vi "ReadCAlexFile.vi"(8 "error in (no error)":errorcluster, 10 "ExpData File Path":path, 11 "CAlexData2":refnum<class "CAlexData2.lvclass">) -> (0 "error out":errorcluster, 3 "CAlexData 2":refnum<class "CAlexData2.lvclass">)   [LabVIEW 2015, in "CAlexData2.lvclass"]
uses:
  CAlexData2.lvclass
  CAlex2/CAlex2.lvclass
  CAlex2/TypeDef/LowerBodyDim.ctl
  CAlexData2.lvclass/CAlexData2.ctl
  ExpData/ExpData.lvclass
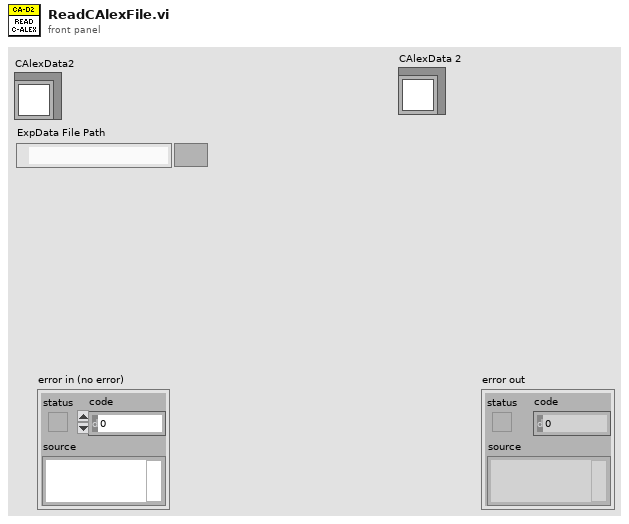
[diagram p1: front panel]
types:
  T1 = typedef "CAlex2.lvclass/LowerBodyDim.ctl" = cluster{"BodyDim(m)":cluster{"ThighLt":dbl, "ShankLt":dbl, "HipWd":dbl}, "BodyWt(kg)":cluster{"Thigh":dbl, "Shank":dbl}, "CuffLoc(m)":cluster{"HipCuffWd":dbl, "HipCuffHt":dbl, "HipCuffFwdShift":dbl, "ThighCuffToKnee":dbl, "ThighCuffDist":dbl, "ShankCuffToKnee":dbl}}
  T2 = cluster{"[0]":dbl, "[1]":dbl, "[2]":dbl, "[3]":dbl, "[4]":dbl, "[5]":dbl}
  T3 = cluster{"array type (2D Dbl)[0]":dbl, "array type (2D Dbl)[1]":dbl, "array type (2D Dbl)[2]":dbl, "array type (2D Dbl)[3]":dbl, "array type (2D Dbl)[4]":dbl, "array type (2D Dbl)[5]":dbl}
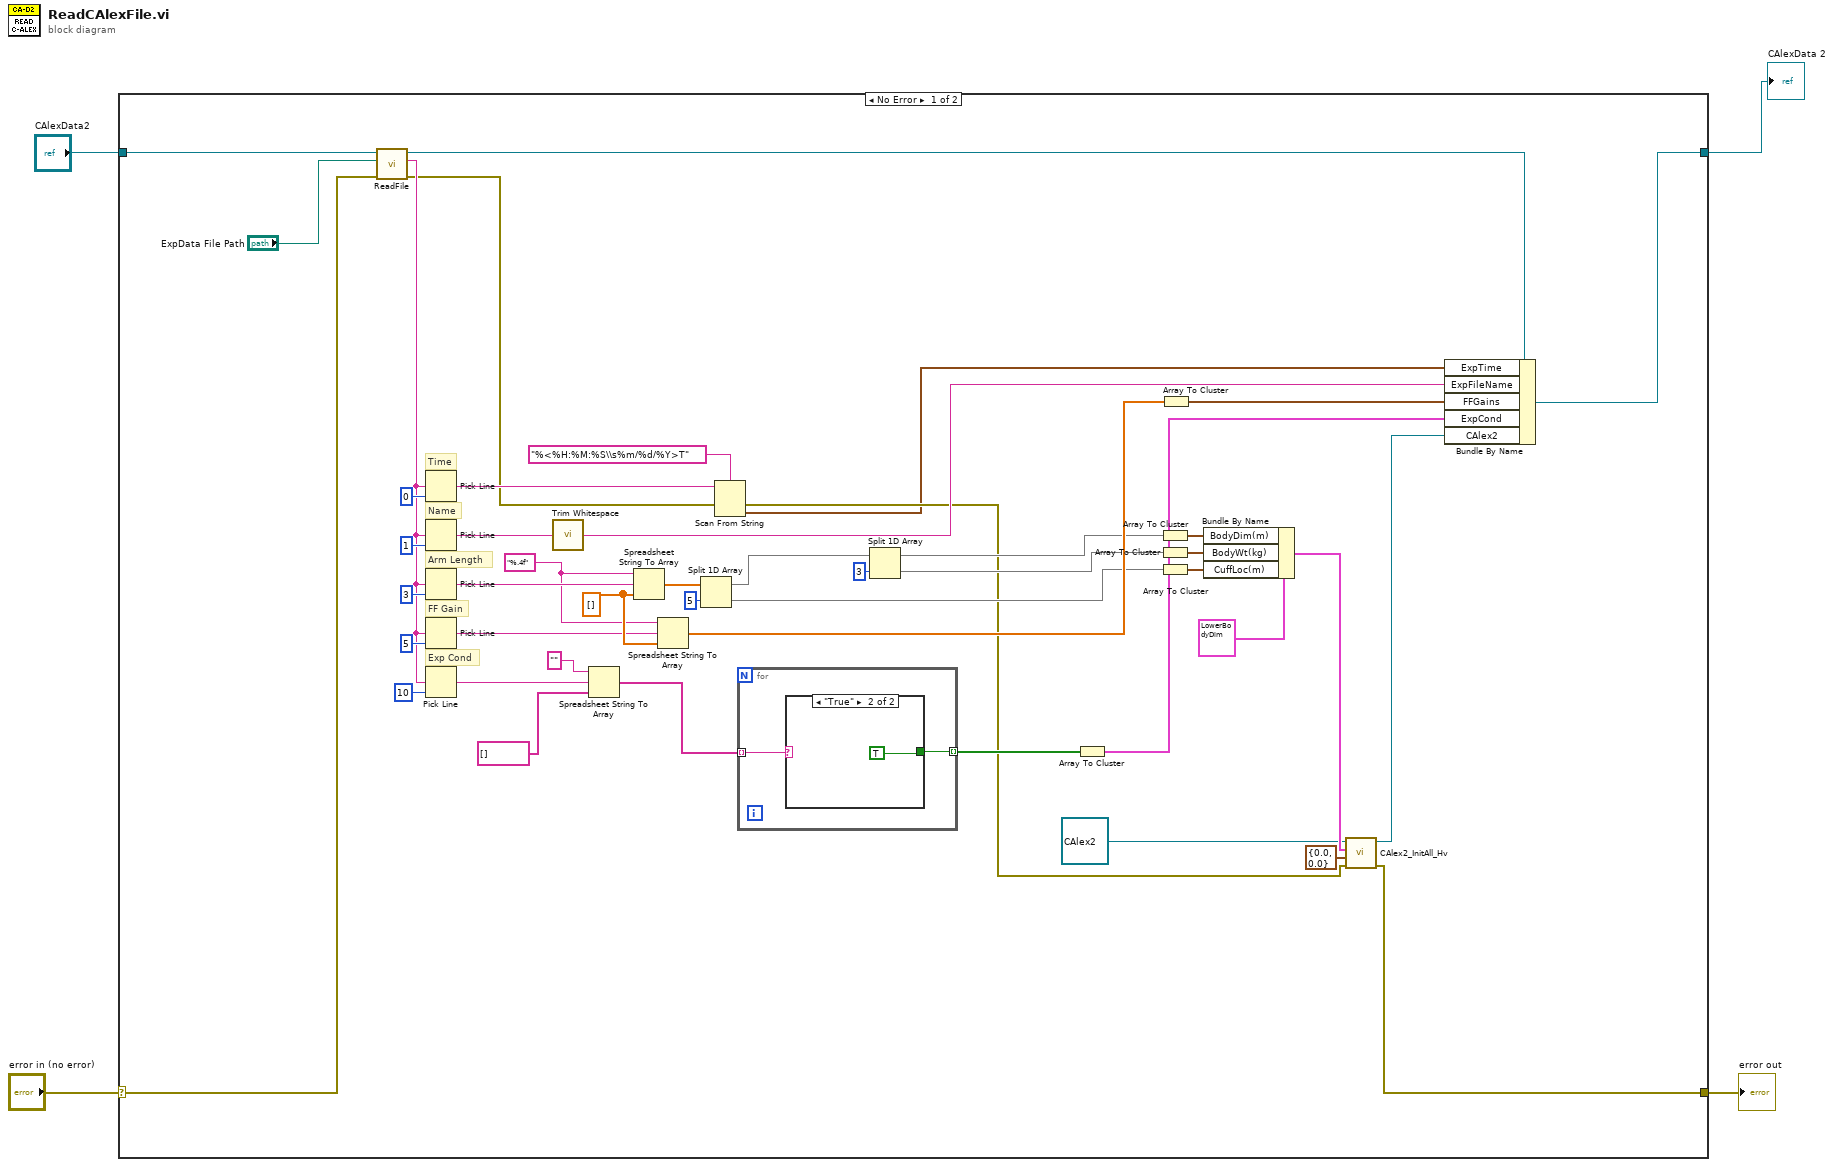
[diagram p0: block diagram]
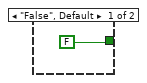
[diagram p2: hidden frame]
diagram:
  n1 = case shown="No Error" "error in (no error)" {
    selector: "error in (no error)" -> [w31 w56]
    tunnel: [w11 w56] -> w3
    tunnel: [w8 w55] -> w1
    tunnel: "CAlexData2" -> [w10 w55]
    frame No Error {
      w35 = "%.4f" ("format (%.3f)")
      w49 = dbl[] [] ("array type (2D Dbl)")
      # "Exp Cond"
      # "FF Gain"
      # "Arm Length"
      # "Name"
      # "Time"
      n2 = call "ReadFile.vi"("error in (no error)"=w31, "ExpData File Path"="ExpData File Path", "ExpData In"=w10) -> ("error out"=w32:errorcluster, "MetaData"=w33:string, "ExpData Out"=w9:refnum<class "CAlexData2.lvclass">)  [unwired: 5 in, 1 out]
      n3 = Pick Line(multi-line string=w33, line index=0) -> (output string=w40:string)  [unwired: 1 in]
      n4 = Pick Line(multi-line string=w33, line index=1) -> (output string=w41:string)  [unwired: 1 in]
      n5 = Pick Line(multi-line string=w33, line index=3) -> (output string=w44:string)  [unwired: 1 in]
      n6 = Pick Line(multi-line string=w33, line index=5) -> (output string=w46:string)  [unwired: 1 in]
      n7 = Pick Line(multi-line string=w33, line index=10) -> (output string=w48:string)  [unwired: 1 in]
      n8 = call <vilib>:"Trim Whitespace.vi"("string"=w41) -> ("trimmed string"=w38:string)  [unwired: 1 in]
      n9 = Spreadsheet String To Array(format string="", spreadsheet string=w48, array type (2D Dbl)=string[] []) -> (array=w21:string[])  [unwired: 1 in]
      n10 = Spreadsheet String To Array(format string=w35, spreadsheet string=w44, array type (2D Dbl)=w49) -> (array=w36:dbl[])  [unwired: 1 in]
      n11 = Spreadsheet String To Array(format string=w35, spreadsheet string=w46, array type (2D Dbl)=w49) -> (array=w30:dbl[])  [unwired: 1 in]
      n12 = Split 1D Array(array=w36, index=5) -> (first subarray=w27:dbl[], second subarray=w24:dbl[])
      n13 = Scan From String(format string="%<%H:%M:%S\\s%m/%d/%Y>T", input string=w40, error in=w32) -> (error out=w12:errorcluster, output 1=w5:timestamp)  [unwired: 2 in, 2 out]
      n14 = for {
        tunnel: w21 -> [w52] mode=indexing
        tunnel: [w51] -> w20 mode=indexing
        n15 = case shown="\"True\"" w52 {
          tunnel: [FALSE TRUE] -> w51
          frame "False", Default {
          }
          frame "True" {
          }
        }
      }
      n16 = Split 1D Array(array=w27, index=3) -> (first subarray=w26:dbl[], second subarray=w25:dbl[])
      n17 = Array To Cluster(array=w20) -> (cluster=w19:cluster{"[0]":bool, "[1]":bool, "[2]":bool})
      n18 = Array To Cluster(array=w26) -> (cluster=w18:cluster{"[0]":dbl, "[1]":dbl, "[2]":dbl})
      n19 = Array To Cluster(array=w25) -> (cluster=w17:cluster{"[0]":dbl, "[1]":dbl})
      n20 = Array To Cluster(array=w24) -> (cluster=w16:T2)
      n21 = Array To Cluster(array=w30) -> (cluster=w29:T3)
      n22 = Bundle By Name(cluster=T1 {"BodyDim(m)"={"ThighLt"=0.0, "ShankLt"=0.0, "HipWd"=0.0}, "BodyWt(kg)"={"Thigh"=0.0, "Shank"=0.0}, "CuffLoc(m)"={"HipCuffWd"=0.0, "HipCuffHt"=0.0, "HipCuffFwdShift"=0.0, "ThighCuffToKnee"=0.0, "ThighCuffDist"=0.0, "ShankCuffToKnee"=0.0}} ("LegProperties"), "BodyDim(m)"=w18, "BodyWt(kg)"=w17, "CuffLoc(m)"=w16) -> (w14:T1)
      n23 = call-dynamic "CAlex2_InitAll_Hv.vi"("error in (no error)"=w12, "ExtraWeight(kg)"=cluster{"Thigh":dbl, "Shank":dbl} {"Thigh"=0.0, "Shank"=0.0}, "LegProperties"=w14, "CAlex2 in"=refnum<class "CAlex2.lvclass"> refnum ("CAlex2")) -> ("error out"=w11:errorcluster, "CAlex2 out"=w15:refnum<class "CAlex2.lvclass">)  [unwired: 6 in]
      n24 = Bundle By Name(cluster=w9, "ExpTime"=w5, "ExpFileName"=w38, "FFGains"=w29, "ExpCond"=w19, "CAlex2"=w15) -> (w8:refnum<class "CAlexData2.lvclass">)
    }
    frame Error {
    }
  }
  "error out" <- w3
  "CAlexData 2" <- w1
